vi "Cal RowNum(SubVI).vi"(9 "EOI":bool, 10 "Last Line Count":i16, 11 "EOL":bool) -> (3 "Output Line Count":i16)   [LabVIEW 2016]
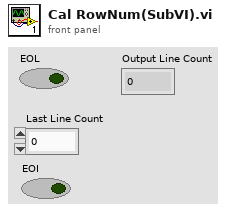
[diagram p1: front panel]
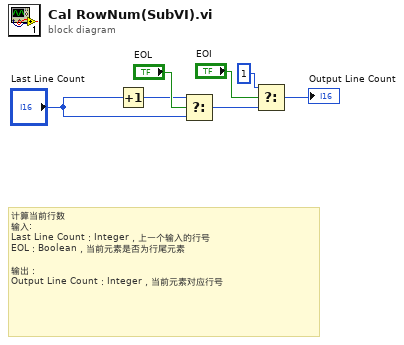
[diagram p0: block diagram]
diagram:
  # "计算当前行数\n输入:\nLast Line Count：Integer，上一个输入的行号\nEOL：Boolean，当前元素是否为行尾元素\n\n输出：\nOutput Line Count：Integer，当前元素对应行号"
  n1 = Increment(x="Last Line Count") -> (x+1=w5:i16)
  n2 = Select(t=w5, s="EOL", f="Last Line Count") -> (s? t:f=w3:i16)
  n3 = Select(t=i16 1, s="EOI", f=w3) -> (s? t:f=→"Output Line Count":i16)
